vi "Splash Screen.vi"() -> ()   [LabVIEW 2021, in "OPC Server AF Launcher.lvlib"]
doc: "This is the top-level VI of this application. When it runs, it behaves like the splash screen many applications use to keep the user occupied while the application loads into memory. This application is quite small, so there is little overhead, which would make the splash screen just flash for a moment. Because that flash is distracting, there is a three-second delay inserted into this VI so that it stays up for a little bit. \n\nThis VI uses a delay-loaded subVI call to load the rest of the application. This trick ensures that the splash screen can load instantly regardless of how large the rest of the VI hierarchy gets, and the loading of the rest of the VIs becomes one step in the load process."
uses:
  OPC Server AF Launcher.lvlib
  OPC Server/OPC Server Actor/Load App.vi
  OPC Server/OPC Server Actor/OPC Server.lvclass
panel:
  out "Waiting Lights":T1
  out "Application Name":string
  out "Current Action":string
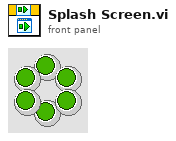
[diagram p1: front panel]
types:
  T1 = cluster{"wait 1":bool, "wait 2":bool, "wait 3":bool, "wait 4":bool, "wait 5":bool, "wait 6":bool}
  T2 = cluster{"[0]":bool, "[1]":bool, "[2]":bool, "[3]":bool, "[4]":bool, "[5]":bool}
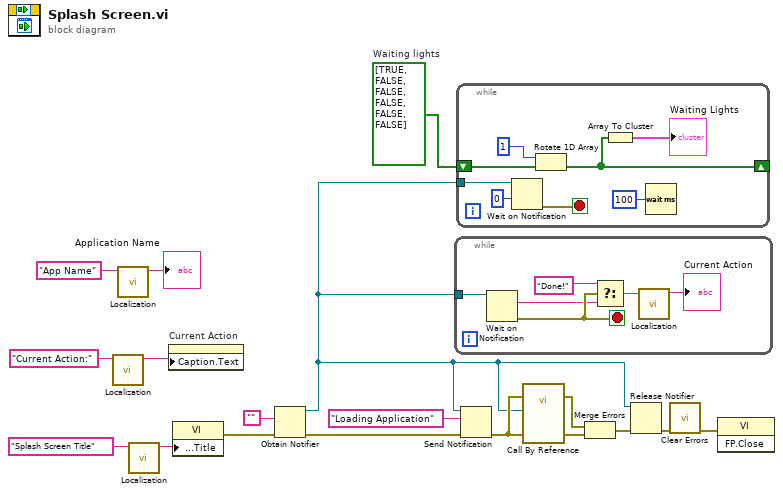
[diagram p0: block diagram]
diagram:
  w8 = bool[] [TRUE, FALSE, FALSE, FALSE, FALSE, FALSE]  # Waiting lights
  n1 = call "Localization.vi"("Unlocalized"="Current Action:" ("Window Title")) -> ("Localized"=w4:string)  [unwired: 10 in]
  n2 = call "Localization.vi"("Unlocalized"="App Name") -> ("Localized"=→"Application Name":string)  [unwired: 10 in]
  n3 = call "Localization.vi"("Unlocalized"="Splash Screen Title" ("Window Title")) -> ("Localized"=w18:string)  [unwired: 10 in]
  n4 = property on="Current Action" class="Str"("Caption.Text"=w4) -> ()  [unwired: 2 in, 2 out]
  n5 = property class="VI"("Front Panel.Title"=w18) -> (error out=w16:errorcluster)  [unwired: 2 in, 1 out]
  n6 = Obtain Notifier(notification data type="", error in (no error)=w16) -> (notifier out=w2:refnum<notifier>, error out=w6:errorcluster)  [unwired: 2 in, 1 out]
  n7 = while {
    tunnel: w2 -> [w23]
    stop <- w22 stop-if-true
    n8 = Wait on Notification(notifier=w23) -> (notification=w20:string, error out=w22:errorcluster)  [unwired: 3 in, 2 out]
    n9 = Select(t="Done!" ("notification"), s=w22, f=w20) -> (s? t:f=w19:string)
    n10 = call "Localization.vi"("Unlocalized"=w19) -> ("Localized"=→"Current Action":string)  [unwired: 10 in]
  }
  n11 = while {
    shift-right: [w26] -> _
    shift-left: w8 -> [w28]
    tunnel: w2 -> [w30]
    stop <- w32 stop-if-true
    n12 = Wait on Notification(notifier=w30, timeout in ms (-1)=0) -> (error out=w32:errorcluster)  [unwired: 2 in, 3 out]
    n13 = Rotate 1D Array(1:w28, 2:1 ("n")) -> (0:w26:bool[])
    n14 = Array To Cluster(array=w26) -> (cluster=→"Waiting Lights":T2)
    n15 = Wait (ms)(milliseconds to wait=u32 100) -> ()  [unwired: 1 out]
  }
  n16 = Send Notification(notification="Loading Application", notifier=w2, error in (no error)=w6) -> (error out=w12:errorcluster)  [unwired: 1 out]
  n17 = call-by-ref "?"(error in=w12, "error in"=w12, "Notifier"=w2) -> (error out=w3:errorcluster, 0:"error out"=w15:errorcluster)  [unwired: 10 in, 1 out]
  n18 = Merge Errors(w3, w15) -> (w1:errorcluster)
  n19 = Release Notifier(notifier=w2, error in (no error)=w1) -> (error out=w14:errorcluster)  [unwired: 1 in, 2 out]
  n20 = call <vilib>:"Clear Errors.vi"("error in (no error)"=w14) -> ("error out"=w7:errorcluster)  [unwired: 5 in, 1 out]
  n21 = invoke class="VI" method="FP.Close"(error in=w7) -> ()  [unwired: 2 in, 3 out]
